vi "Set Entry Mode.vi"(6 "chip select (1st chip)":enum16{"1st chip", "2nd chip"}(ring), 8 "error in (no error)":errorcluster, 10 "entry mode":T1(ring), 11 "LCD in":u32) -> (0 "error out":errorcluster, 3 "LCD out":u32)   [LabVIEW 2015, in "HD44780 FPGA.lvlib"]
doc: "Sets the entry mode of character LCD devices. The entry mode defines the cursor moving direction and display shifting direction after a read data or write data operation."
uses:
  <vilib>/EmbeddedDisplay/Hitachi HD44780/FPGA/HD44780 FPGA.lvlib
  <vilib>/EmbeddedDisplay/Hitachi HD44780/Common/HD44780 Common.lvlib
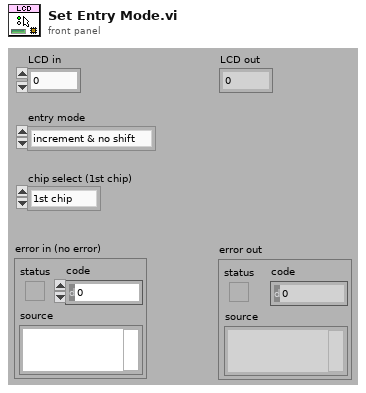
[diagram p1: front panel]
types:
  T1 = enum8{"increment & no shift", "increment & shift", "decrement & no shift", "decrement & shift"}
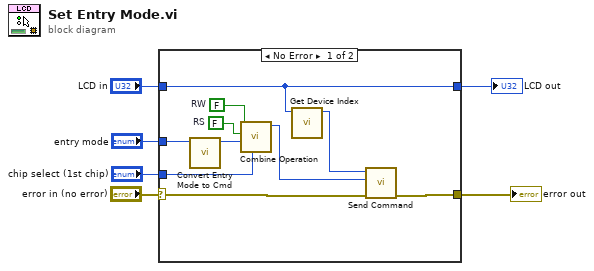
[diagram p0: block diagram]
diagram:
  n1 = case shown="No Error" "error in (no error)" {
    selector: "error in (no error)" -> [w11 w17]
    tunnel: "entry mode" -> [w16 _]
    tunnel: "chip select (1st chip)" -> [w15 _]
    tunnel: "LCD in" -> [w7 w18]
    tunnel: [w7 w18] -> w2
    tunnel: [w12 w17] -> w1
    frame No Error {
      w9 = FALSE  # RW
      w10 = FALSE  # RS
      n2 = call <vilib>:"Convert Entry Mode to Cmd.vi"("entry mode"=w16) -> ("Numeric"=w14:u8)  [unwired: 10 in]
      n3 = call <vilib>:"Combine Operation.vi"("chip select  (1st chip)"=w15, "cmd/data (0)"=w14, "RS"=w10, "R/W"=w9) -> ("output"=w13:u32)  [unwired: 7 in]
      n4 = call <vilib>:"Get Device Index.vi"("LCD in"=w7) -> ("device index"=w8:i8)  [unwired: 10 in]
      n5 = call <vilib>:"Send Command.vi"("error in (no error)"=w11, "operation"=w13, "device index"=w8) -> ("error out"=w12:errorcluster)  [unwired: 6 in, 2 out]
    }
    frame Error {
    }
  }
  "LCD out" <- w2
  "error out" <- w1
